vi "GetProgramDirectory.vi"(8 "error in":errorcluster, 10 "PathName":string="\\", 11 "VISA resource name":refnum<visa-resource-name>) -> (0 "error out":errorcluster, 2 "Program Directory":string, 3 "VISA resource name out":refnum<visa-resource-name>)   [LabVIEW 2023, in "Thermotron 8800.lvlib"]
doc: "DIRP\nCommand name: Send program directory\nCommand type: Programming\nDescription: This command queries a specific directory on the 8800 for a list of program files and directories. This command will return the name of the program or directory followed\nby a number. If the name refers to a program file, the number will be the number of\nintervals in the program. If the name refers to a directory, the number will be -2.\nContinue calling this command to get a list of all directories and programs on the\n8800. When you have iterated through all the items in the current directory this\ncommand will return “No More Files” for the name and -1 for the number.\n\nSyntax: DIRPpathname?\nWhere:\npathname is the name of a path on the 8800 or “\\” for the root path of the 8800.\n\nQuery example 1: DIRP\\?\n8800 response: humidity test, 5 (program called humidity test with five intervals)\n\nQuery example 2: DIRP\\?\n8800 response: Pre-programmed Tests, -2 (directory called Pre-programmed Tests)\n\nQuery example 3: DIRP\\Pre-programmed Tests?\n8800 response: 8800-SE humidity, 6 (program called 8800-SE humidity with six intervals)\n\nQuery example 4: DIRP\\Pre-programmed Tests?\n8800 response: No More Files, -1 (You have iterated through all the items in the Pre-programmed Tests directory.)"
uses:
  Thermotron 8800.lvlib
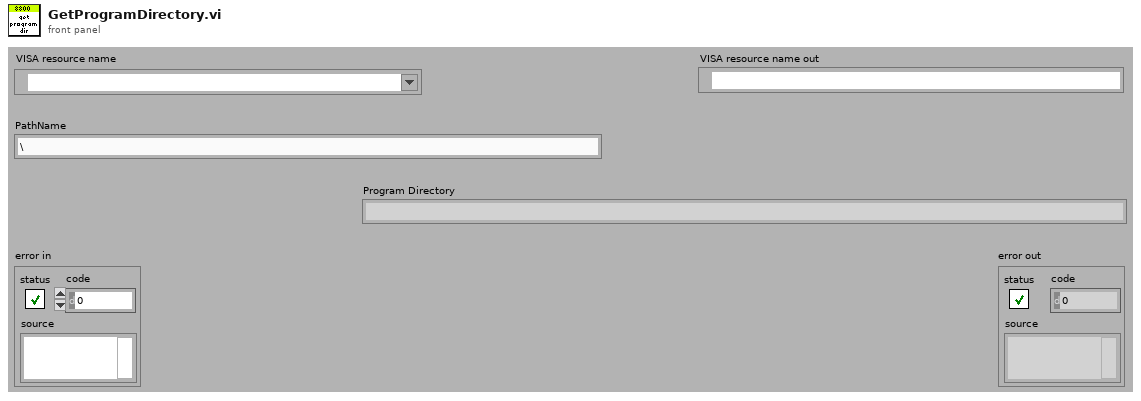
[diagram p1: front panel]
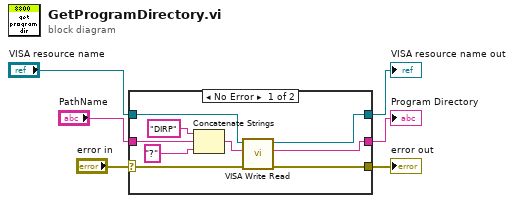
[diagram p0: block diagram]
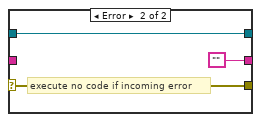
[diagram p2: hidden frame]
diagram:
  n1 = case shown="No Error" "error in" {
    selector: "error in" -> [w12 w17]
    tunnel: [w9 w18] -> w5
    tunnel: "VISA resource name" -> [w10 w18]
    tunnel: [w11 w17] -> w3
    tunnel: "PathName" -> [w8 _]
    tunnel: [w7 ""] -> w1
    frame No Error {
      n2 = Concatenate Strings("DIRP" ("8800 Command"), w8, "?" ("8800 Command")) -> (w13:string)
      n3 = call "VISA Write Read.vi"("error in (no error)"=w12, "8800 Command"=w13, "VISA Refnum in"=w10) -> ("error out"=w11:errorcluster, "read buffer"=w7:string, "VISA Refnum out"=w9:refnum<visa-resource-name>)  [unwired: 6 in]
    }
    frame Error {
      # "execute no code if incoming error"
    }
  }
  "VISA resource name out" <- w5
  "error out" <- w3
  "Program Directory" <- w1
